vi "GetRectUnionFloat.vi"(8 "No Error":errorcluster, 10 "B":T1, 11 "A":T1) -> (0 "Error Out":errorcluster, 3 "Union":T1)   [LabVIEW 2026, in "SDL3.lvlib" / "Rect.lvlib"]
doc: "<B>Summary</B>\nCalculate the union of two rectangles with float precision."
uses:
  Rect.lvlib
  FRect--cluster.ctl
  <vilib>/Utility/error.llb/Error Cluster From Error Code.vi
  Error/Error.lvlib
  Lib/SDL3.dll
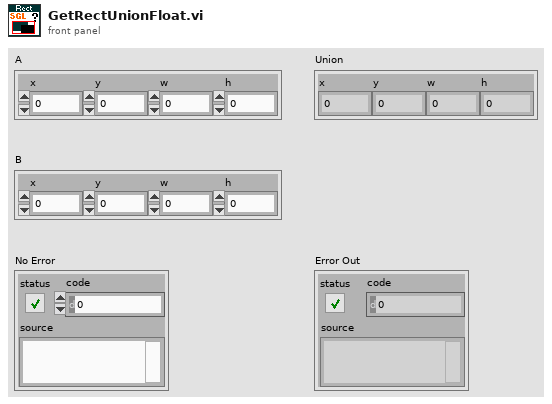
[diagram p1: front panel]
types:
  T1 = typedef "SDL3.lvlib/Rect.lvlib/FRect--cluster.ctl" = cluster{"x":sgl, "y":sgl, "w":sgl, "h":sgl}
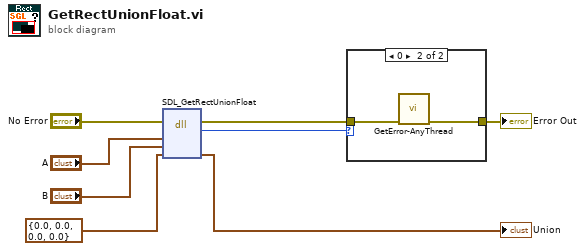
[diagram p0: block diagram]
diagram:
  n1 = dll-call lib="C:/Users/saukko/Dev/LV-SDL3/Sources/SDL3/Lib/SDL3.*" fn="SDL_GetRectUnionFloat"(error in="No Error", "A"="A", "B"="B", "result"=T1 {"x"=0.0, "y"=0.0, "w"=0.0, "h"=0.0} ("B")) -> (error out=w2:errorcluster, "return type"=w1:i32, "result"=→"Union":T1)  [unwired: 4 in, 1 out]
  n2 = case shown="0" w1 {
    tunnel: w2 -> [w9 w11]
    tunnel: [w9 w10] -> w4
    frame Default {
    }
    frame 0 {
      n3 = call "GetError-AnyThread.vi"("No Error"=w11) -> ("Error Out"=w10:errorcluster)  [unwired: 10 in]
    }
  }
  "Error Out" <- w4
